vi "Pre Launch Init.vi"(11 "Software Lock-in in":refnum<class "Software Lock-in.lvclass">) -> (0 "error out":errorcluster, 3 "Software Lock-in out":refnum<class "Software Lock-in.lvclass">)   [LabVIEW 2015, in "Software Lock-in.lvclass"]
doc: "(<B>Filename</B>: Actor Framework.lvlib:Actor.lvclass:Pre Launch Init.vi)\n\nDefines behavior that occurs after the Launch Actor method is invoked but before the actor's Actor Core method begins running.\n\nThe Pre Launch Init method is guaranteed to finish before the Launch Actor method returns to its caller and before the actor itself receives any messages. Any references that the Pre Launch Init method obtains are guaranteed to have the same lifetime as the actor itself. Any errors that the Pre Launch Init method returns will abort the launch.\n\nBy default, this method does nothing. A descendant class may override it to define behavior."
uses:
  Software Lock-in.lvclass
  Lock-in modulation.ctl
  Software Lock-in.lvclass/Software Lock-in.ctl
  Mag Lab Hardware.lvclass
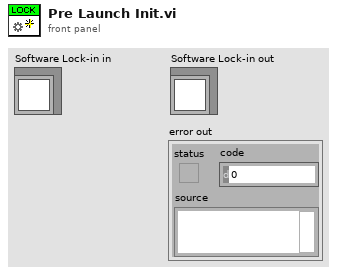
[diagram p1: front panel]
types:
  T1 = typedef "Lock-in modulation.ctl" = cdb[]
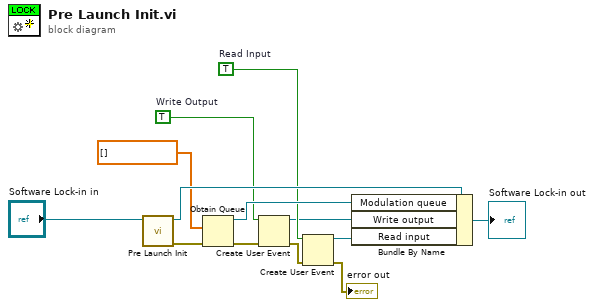
[diagram p0: block diagram]
diagram:
  w4 = TRUE  # Read Input
  w7 = TRUE  # Write Output
  n1 = call-parent "Pre Launch Init.vi"("Mag Lab Hardware in"="Software Lock-in in") -> ("error out"=w11:errorcluster, "Mag Lab Hardware out"=w13:refnum<class "Software Lock-in.lvclass">)  [unwired: 9 in]
  n2 = Obtain Queue(element data type=T1 [] ("Lock-in modulation"), error in (no error)=w11) -> (queue out=w8:refnum<queue>, error out=w6:errorcluster)  [unwired: 3 in, 1 out]
  n3 = Create User Event(user event datatype=w7, error in=w6) -> (user event=w3:refnum<user-event>, error out=w5:errorcluster)
  n4 = Create User Event(user event datatype=w4, error in=w5) -> (user event=w2:refnum<user-event>, error out=→"error out":errorcluster)
  n5 = Bundle By Name(cluster=w13, "Modulation queue"=w8, "Write output"=w3, "Read input"=w2) -> (→"Software Lock-in out":refnum<class "Software Lock-in.lvclass">)
